vi "_Read_T.vi"(8 "error in (no error)":errorcluster, 10 "First Query?":bool, 11 "Postgres Connector In":refnum<class "Postgres Connector.lvclass">) -> (0 "error out":errorcluster, 3 "Postgres Connector Out":refnum<class "Postgres Connector.lvclass">)   [LabVIEW 2019, in "PG_LIB.lvlib" / "Postgres Connector.lvclass"]
doc: "This VI is used to decode the first part of message the database send after a query. It shouls start with the \"RowDescription\" and the first letter should be \"T\". Knowing that, we can wait util the letter show up and that way, consider we have received the response."
uses:
  Postgres Connector.lvclass
  Cluster_Reader_Infos.ctl
  Enum_RowDescription_State_Machine.ctl
  Postgres Connector.lvclass/Postgres Connector.ctl
panel:
  out "RowDescription":string
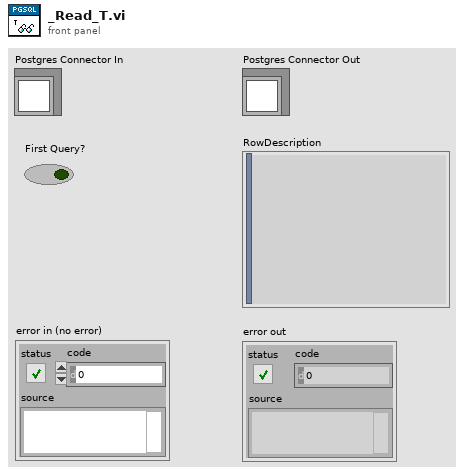
[diagram p1: front panel]
types:
  T1 = typedef "PG_LIB.lvlib/Postgres Connector.lvclass/Cluster_Reader_Infos.ctl" = cluster{"Byte Length":i32}
  T2 = typedef "PG_LIB.lvlib/Postgres Connector.lvclass/Enum_RowDescription_State_Machine.ctl" = enum16{"Check For Error", "Wait For T", "Wait For D", "Wait For Z", "C Byte Length", "Z Byte Length", "n Byte Length", "Byte Length", "Get Infos", "Check For End", "Flush", "Quit"}
  T3 = enum16{"Standard", "Buffered", "CRLF", "Immediate"}
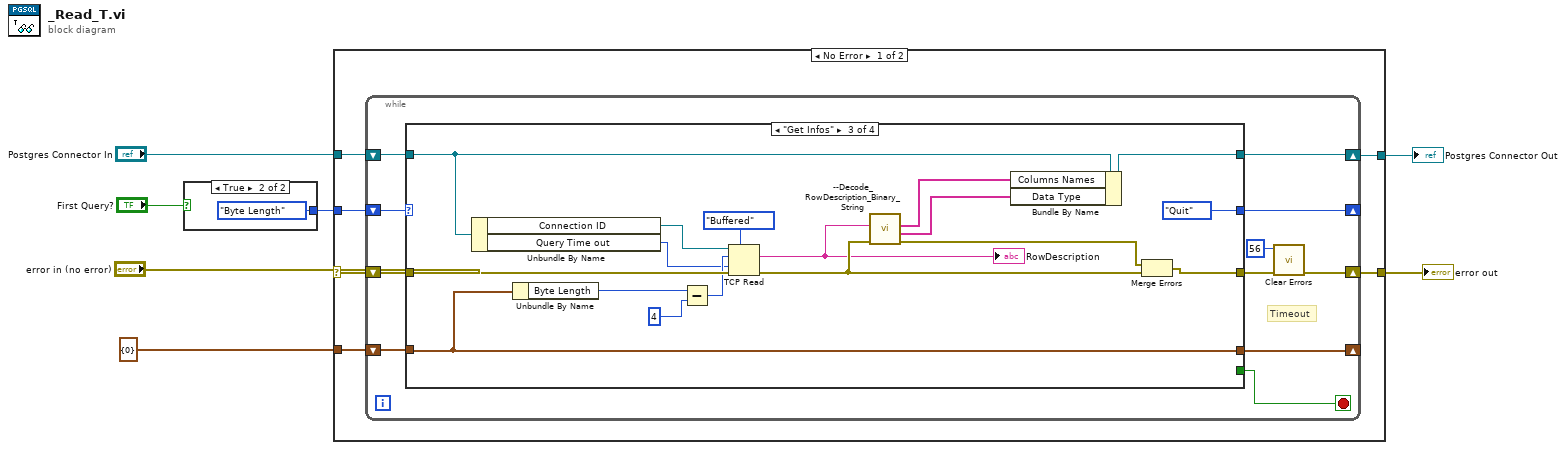
[diagram p0: block diagram]
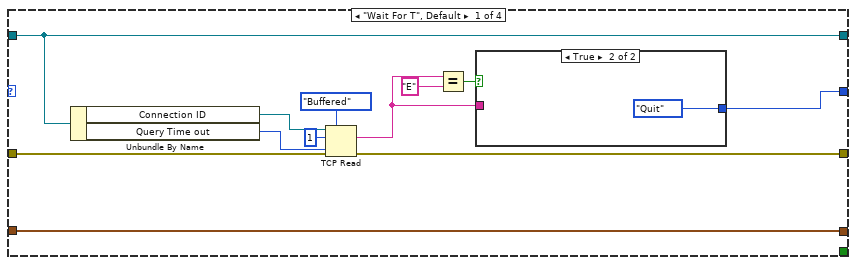
[diagram p2: hidden frame]
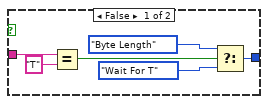
[diagram p3: hidden frame]
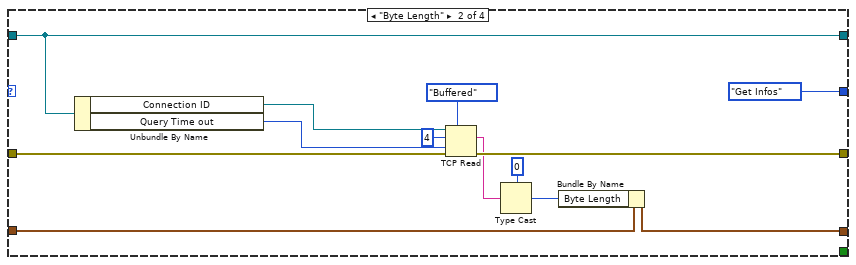
[diagram p4: hidden frame]
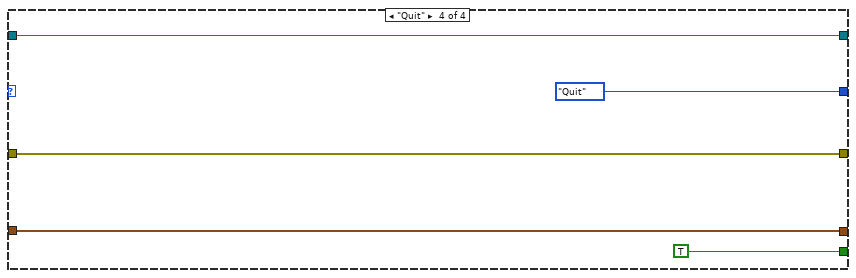
[diagram p5: hidden frame]
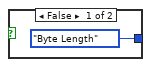
[diagram p7: hidden frame]
diagram:
  n1 = case shown="True" "First Query?" {
    tunnel: [Enum_RowDescription_State_Machine."Byte Length" Enum_RowDescription_State_Machine."Byte Length"] -> w6
    frame False {
    }
    frame True {
    }
  }
  n2 = case shown="No Error" "error in (no error)" {
    selector: "error in (no error)" -> [w14 w82]
    tunnel: "Postgres Connector In" -> [w15 w81]
    tunnel: w6 -> [w13 _]
    tunnel: [w12 w82] -> w5
    tunnel: T1 {"Byte Length"=0} ("Reader_Infos") -> [w11 _]
    tunnel: [w10 w81] -> w1
    frame No Error {
      n3 = while {
        shift-right: [w22] -> w12
        shift-left: w14 -> [w25]
        shift-right: [w20] -> _
        shift-left: w13 -> [w24]
        shift-right: [w18] -> _
        shift-left: w11 -> [w19]
        shift-right: [w16] -> w10
        shift-left: w15 -> [w26]
        stop <- w17 stop-if-true
        # "Timeout"
        n4 = case shown="\"Get Infos\"" w24 {
          tunnel: w26 -> [w28 w55 w63 w76]
          tunnel: w25 -> [w35 w54 w73 w79]
          tunnel: [w34 w53 w67 w79] -> w23
          tunnel: [w33 Enum_RowDescription_State_Machine."Get Infos" Enum_RowDescription_State_Machine."Quit" Enum_RowDescription_State_Machine."Quit"] -> w20
          tunnel: w19 -> [w32 w48 w71 w80]
          tunnel: [w32 w47 w71 w80] -> w18
          tunnel: [_ _ _ TRUE] -> w17
          tunnel: [w28 w55 w62 w76] -> w16
          frame "Wait For T", Default {
            n5 = Unbundle By Name(w28) -> ("Connection ID"=w37:refnum<k5>, "Query Time out"=w27:i32)
            n6 = TCP Read(connection ID=w37, bytes to read=1, error in (no error)=w35, 7:T3."Buffered" ("mode (standard)"), 9:w27) -> (data out=w30:string, error out=w34:errorcluster)  [unwired: 1 out]
            n7 = Equal?(x=w30, y="E") -> (x = y?=w29:bool)
            n8 = case shown="True" w29 {
              tunnel: [w42 Enum_RowDescription_State_Machine."Quit"] -> w33
              tunnel: w30 -> [w39 _]
              frame False {
                n9 = Equal?(x=w39, y="T") -> (x = y?=w43:bool)
                n10 = Select(t=Enum_RowDescription_State_Machine."Byte Length", s=w43, f=Enum_RowDescription_State_Machine."Wait For T") -> (s? t:f=w42:T2)
              }
              frame True {
              }
            }
          }
          frame "Byte Length" {
            n11 = Unbundle By Name(w55) -> ("Connection ID"=w57:refnum<k5>, "Query Time out"=w46:i32)
            n12 = TCP Read(connection ID=w57, bytes to read=4, error in (no error)=w54, 7:T3."Buffered" ("mode (standard)"), 9:w46) -> (data out=w51:string, error out=w53:errorcluster)  [unwired: 1 out]
            n13 = Type Cast(type=0, x=w51) -> (*(type *) &x=w50:i32)
            n14 = Bundle By Name(cluster=w48, "Byte Length"=w50) -> (w47:T1)
          }
          frame "Get Infos" {
            n15 = Unbundle By Name(w63) -> ("Connection ID"=w74:refnum<k5>, "Query Time out"=w59:i32)
            n16 = Unbundle By Name(w71) -> ("Byte Length"=w70:i32)
            n17 = Subtract(x=w70, y=4 ("bytes to read")) -> (x-y=w69:i32)
            n18 = TCP Read(connection ID=w74, bytes to read=w69, error in (no error)=w73, 7:T3."Buffered" ("mode (standard)"), 9:w59) -> (data out=w65:string, error out=w66:errorcluster)  [unwired: 1 out]
            "RowDescription" <- w65
            n19 = call "--Decode_RowDescription_Binary_String.vi"("error in (no error)"=w66, "binary string"=w65) -> ("error out"=w64:errorcluster, "Data Type"=w60:string[], "Column Names"=w61:string[])  [unwired: 7 in]
            n20 = Bundle By Name(cluster=w63, "Columns Names"=w61, "Data Type"=w60) -> (w62:refnum<class "Postgres Connector.lvclass">)
            n21 = Merge Errors(w64, w66) -> (w67:errorcluster)
          }
          frame "Quit" {
          }
        }
        n22 = call <vilib>:"Clear Errors.vi"("error in (no error)"=w23, "specific error code to clear (0: all)"=56) -> ("error out"=w22:errorcluster)  [unwired: 4 in, 1 out]
      }
    }
    frame Error {
    }
  }
  "error out" <- w5
  "Postgres Connector Out" <- w1
